vi "S2C_FORNAX_Poly_SystemSettingsCommand.vi"(8 "Error In":errorcluster, 10 "SystemSettingsCommand":T3={"Partition"="Default", "Message"="SystemSettingsCommand", "M_SystemSetting"=0, "M_Command"=0, "M_IntValue"=0, "M_StringValue"=""} {"M_Command" items=["SYSTEM_SETTINGS_COMMAND_NONE", "SYSTEM_SETTINGS_COMMAND_WRITE", "SYSTEM_SETTINGS_COMMAND_READ", "SYSTEM_SETTINGS_COMMAND_RESTORE_TO_DEFAULT"]; "M_SystemSetting" items=["SYSTEM_SETTINGS_INVALID", "SYSTEM_SETTINGS_COUNTRY", "SYSTEM_SETTINGS_REGION", "SYSTEM_SETTINGS_BIPOLAR_RESECTION", "SYSTEM_SETTINGS_INSTRUMENT_ID_MODE", "SYSTEM_SETTINGS_SMOKE_EVAC_MODE", "NUM_SYSTEM_SETTINGS"]}, 11 "Settings":T4={"Driver"="Fornax", "Command"="SystemSettingsCommand", "Return"="ErrorStatus", "Parameters"="", "Timeout"=10.0}) -> (0 "Error Out":errorcluster, 3 "Response":string)   [LabVIEW 2015]
uses:
  Typedefs/SystemSettings.ctl
  Typedefs/SystemSettingsCommand.ctl
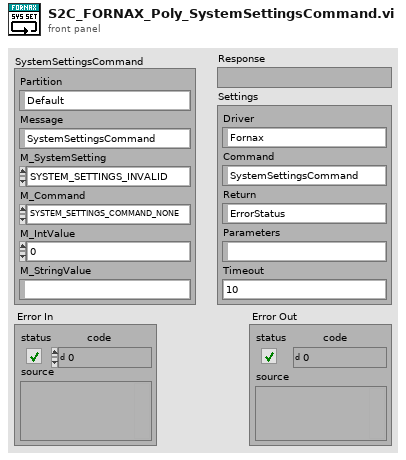
[diagram p1: front panel]
types:
  T1 = typedef "SystemSettings.ctl" = i16
  T2 = typedef "SystemSettingsCommand.ctl" = i16
  T3 = cluster{"Partition":string, "Message":string, "M_SystemSetting":T1, "M_Command":T2, "M_IntValue":i32, "M_StringValue":string}
  T4 = cluster{"Driver":string, "Command":string, "Return":string, "Parameters":string, "Timeout":dbl}
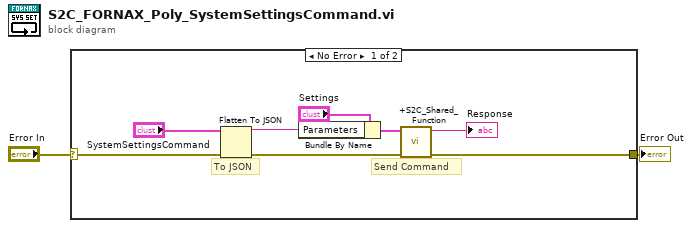
[diagram p0: block diagram]
diagram:
  n1 = case shown="No Error" "Error In" {
    selector: "Error In" -> [w6 w11]
    tunnel: [w5 w11] -> w1
    frame No Error {
      # "To JSON"
      # "Send Command"
      n2 = Flatten To JSON(anything="SystemSettingsCommand", error in (no error)=w6) -> (JSON string=w7:string, 11:w9:errorcluster)  [unwired: 1 in]
      n3 = Bundle By Name(cluster="Settings", "Parameters"=w7) -> (w10:T4)
      n4 = call "+S2C_Shared_Function.vi"("Error In"=w9, "Settings"=w10) -> ("Error Out"=w5:errorcluster, "Response"=→"Response":string)  [unwired: 8 in]
    }
    frame Error {
    }
  }
  "Error Out" <- w1
